vi "Connect.vi"(8 "error in":errorcluster, 11 "MiniIO in":refnum<class "MiniIO.lvclass">) -> (0 "error out":errorcluster, 3 "MiniIO out":refnum<class "MiniIO.lvclass">)   [LabVIEW 2018, in "MiniIO.lvlib" / "MiniIO.lvclass"]
uses:
  MiniIO.lvclass
  MiniIO.lvclass/MiniIO.ctl
  <vilib>/NI/Modbus Library/API/Wrapper/Create Serial Master.vi
  <vilib>/NI/Modbus Library/API/Wrapper/API Main.lvlib
  PPLs/PLC/Parent/PLC.lvlibp/PLC.lvclass
  C:/AME Test Engineering/LabVIEW/PPLs/PLC/Parent/PLC.lvlibp/PLC.lvclass
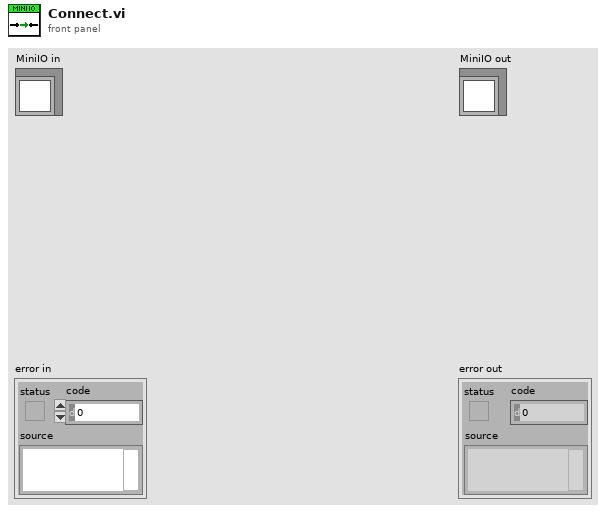
[diagram p1: front panel]
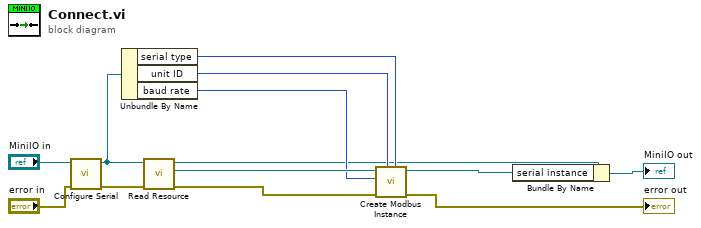
[diagram p0: block diagram]
diagram:
  n1 = call "Configure Serial.vi"("error in"="error in", "MiniIO in"="MiniIO in") -> ("error out"=w6:errorcluster, "MiniIO out"=w7:refnum<class "MiniIO.lvclass">)  [unwired: 8 in]
  n2 = Unbundle By Name(w7) -> ("serial type"=w4:enum16{"RTU", "ASCII"}, "unit ID"=w3:u8, "baud rate"=w2:u32)
  n3 = call "Read Resource.vi"("error in (no error)"=w6, "PLC in"=w7) -> ("error out"=w5:errorcluster, "Resource"=w8:refnum<visa-resource-name>, "PLC out"=w1:refnum<class "MiniIO.lvclass">)  [unwired: 7 in]
  n4 = call-poly <vilib>:"Create Modbus Instance.vi"("serial type"=w4, "unit ID"=w3, "error in"=w5, "baud rate"=w2, "VISA resource name"=w8) -> ("error out"=→"error out":errorcluster, "serial master instance"=w12:refnum<class "Modbus Master.lvclass">)  [unwired: 5 in]
  n5 = Bundle By Name(cluster=w1, "serial instance"=w12) -> (→"MiniIO out":refnum<class "MiniIO.lvclass">)
